vi "SVPO Analog Tacho Process.vi"   [LabVIEW 2017, in "SoundVib_TachProcess.lvlib"]
doc: "Locates tachometer pulse positions in analog tachometer signals using the number of generated pulses per revolution, the pulse width, and the arrival edge of the tachometer pulse. Use this VI on embedded targets that have limited computational resources. Wire data to the <B>analog tacho signal</B> input to determine the polymorphic instance to use or manually select the instance."
uses:
  <vilib>/addons/Sound and Vibration/Order Analysis/Tach Process/SoundVib_TachProcess.lvlib
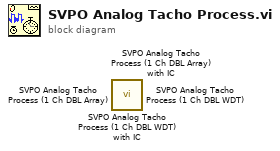
[diagram p0: block diagram]
diagram:
  n1 = call <vilib>:"SVPO Analog Tacho Process (1 Ch DBL WDT) with IC.vi"() -> ()  [unwired: 13 in, 3 out]
  n2 = call <vilib>:"SVPO Analog Tacho Process (1 Ch DBL Array) with IC.vi"() -> ()  [unwired: 13 in, 3 out]
  n3 = call <vilib>:"SVPO Analog Tacho Process (1 Ch DBL Array).vi"() -> ()  [unwired: 14 in, 2 out]
  n4 = call <vilib>:"SVPO Analog Tacho Process (1 Ch DBL WDT).vi"() -> ()  [unwired: 14 in, 2 out]
